vi "String IP to U32.vi"(11 "String IP":string) -> (3 "U32 IP":u32 format="%.0x")   [LabVIEW 2020]
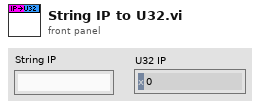
[diagram p1: front panel]
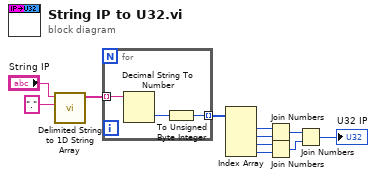
[diagram p0: block diagram]
diagram:
  n1 = call <vilib>:"Delimited String to 1D String Array.vi"("delimiter"=".", "delimited string"="String IP") -> ("string array"=w9:string[])  [unwired: 9 in]
  n2 = for {
    tunnel: w9 -> [w14] mode=indexing
    tunnel: [w12] -> w8 mode=indexing
    n3 = Decimal String To Number(string=w14) -> (number=w13:i32)  [unwired: 2 in, 1 out]
    n4 = To Unsigned Byte Integer(number=w13) -> (unsigned 8bit integer=w12:u8)
  }
  n5 = Index Array(array=w8) -> (element #1=w7:u8, element #2=w6:u8, element #3=w5:u8, element #4=w4:u8)  [unwired: 4 in]
  n6 = Join Numbers(hi=w7, lo=w6) -> ((hi.lo)=w3:u16)
  n7 = Join Numbers(hi=w5, lo=w4) -> ((hi.lo)=w2:u16)
  n8 = Join Numbers(hi=w3, lo=w2) -> ((hi.lo)=→"U32 IP":u32)
